vi "ReadFromFile.vi"(8 "error in (no error)":errorcluster, 11 "Temporary File Path in":path) -> (0 "error out":errorcluster, 2 "File content":string, 3 "Temporary File Path out":path)   [LabVIEW 2014, in "MassCompile.lvclass"]
uses:
  MassCompile.lvclass
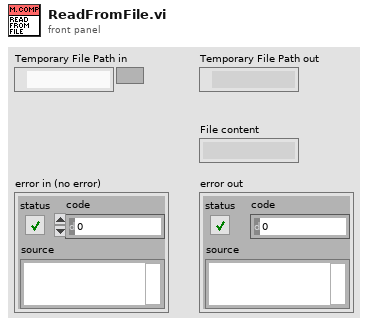
[diagram p1: front panel]
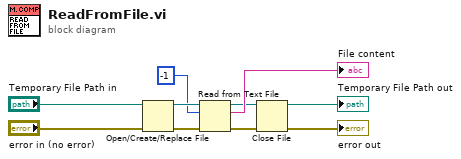
[diagram p0: block diagram]
diagram:
  n1 = Open/Create/Replace File(file path (use dialog)="Temporary File Path in", error in="error in (no error)") -> (refnum out=w5:refnum<file>, error out=w4:errorcluster)  [unwired: 4 in, 1 out]
  n2 = Read from Text File(file (use dialog)=w5, count=-1, error in=w4) -> (refnum out=w7:refnum<file>, text=→"File content":string, error out=w6:errorcluster)  [unwired: 1 in, 1 out]
  n3 = Close File(refnum=w7, error in=w6) -> (path=→"Temporary File Path out":path, error out=→"error out":errorcluster)
